vi "Create.vi"(8 "error in":errorcluster, 10 "ICommunicate":refnum<class "ICommunicate.lvclass">) -> (0 "error out":errorcluster, 3 "Network Management out":refnum<class "Network Management.lvclass">)   [LabVIEW 2020, in "CANopen.lvlib" / "Network Management.lvlib" / "Network Management.lvclass"]
uses:
  Network Management.lvclass
  Network Management.lvclass/Network Management.ctl
  HAL/Source/Interfaces/ICommunicate/ICommunicate.lvclass
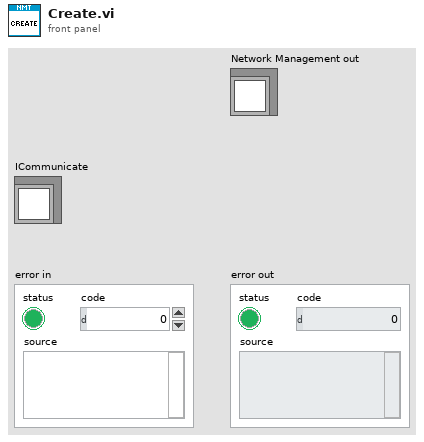
[diagram p1: front panel]
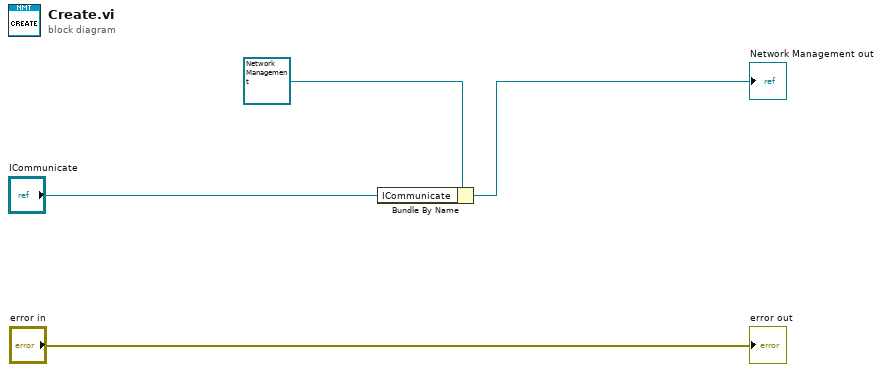
[diagram p0: block diagram]
diagram:
  n1 = Bundle By Name(cluster=refnum<class "Network Management.lvclass"> refnum ("Network Management out"), "ICommunicate"="ICommunicate") -> (→"Network Management out":refnum<class "Network Management.lvclass">)
  "error out" <- "error in"
